vi "TAT_PLC_Data_read_BOLLEAN_St2.vi"(7 "Enum":enum16{"Read", "Write"}(ring), 8 "error in (no error)":errorcluster, 10 "Array":bool[](array[boolean])) -> (0 "error out":errorcluster, 2 "Array 2":bool[](array[boolean]))   [LabVIEW 2017]
panel:
  # "STATION 2"
  # "SCAN BYPASS---2598\nRQS TO TCO READ SCAN DATA \n\nCYCLE START (RUNNING CYCLE)\nCYCLE STOP\nCYCLE COMPLETE\nby pass station 1 Bit --45325\nStation 1 valid BIT\nPOWER FOLD CURENT M603---2651\nGLASS ACTUATOR CURANT 1 MA\nGLASS ACTUATOR CURANT 2 MA\n\n\nGLASS PUL TEST\nSKY \nGROUND\nINTERNAL(DEG)\nEXTERNAL(DEG)\n GASKET PRESENT SENSOR 1 D1811\n GASKET PRESENT SENSOR 2\n PY1B & HBC LH PART VERIFICATION SENSOR\n PY1B & HBC RH PART VERIFICATION SENSOR\n PY1B LHD RH PART SENSOR\n PY1B LHD LH PART SENSOR\n RAREJECTION BIN\n PRINT LABEL PICKUP"
  # "CONTROL PROCESS TO  LABVIEW from PLC"
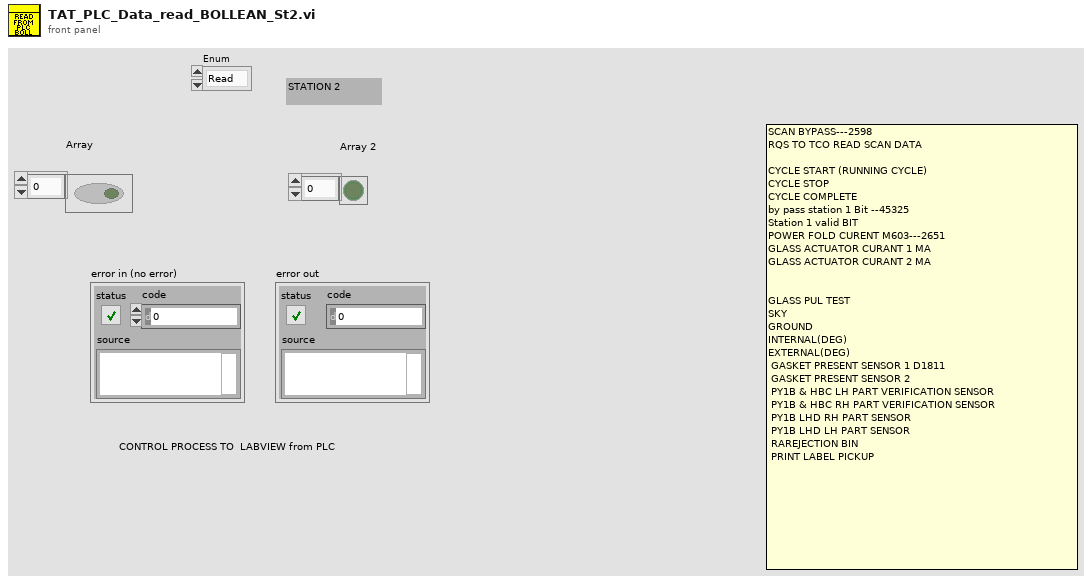
[diagram p1: front panel]
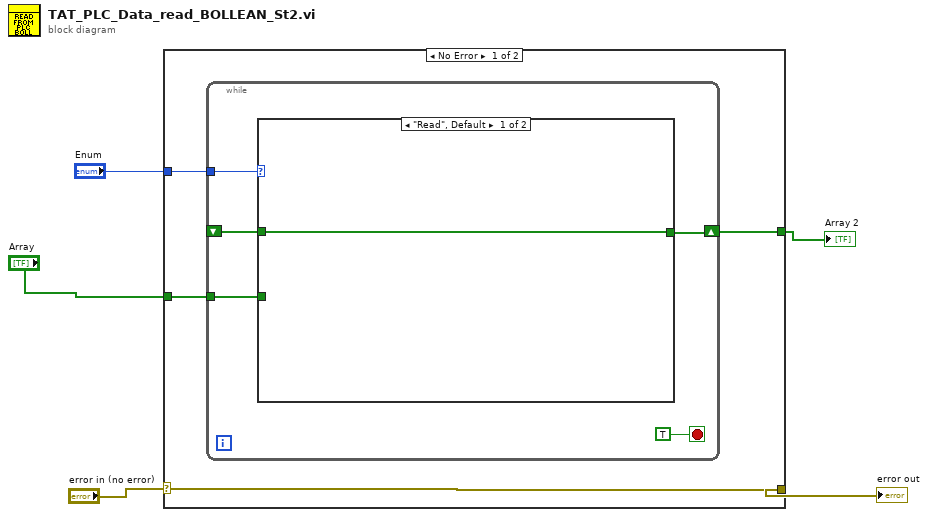
[diagram p0: block diagram]
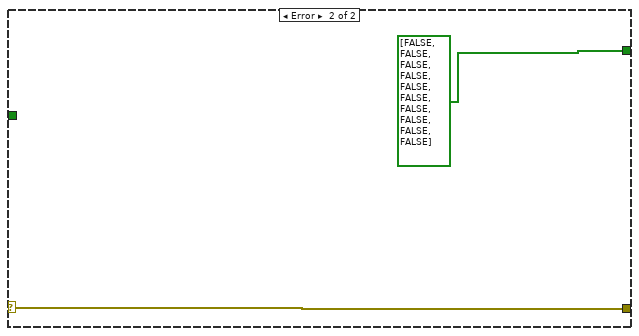
[diagram p3: hidden frame]
diagram:
  n1 = case shown="No Error" "error in (no error)" {
    selector: "error in (no error)" -> [w6 w18]
    tunnel: [w6 w18] -> w5
    tunnel: "Enum" -> [w9 _]
    tunnel: "Array" -> [w8 _]
    tunnel: [w7 bool[] [FALSE, FALSE, FALSE, FALSE, FALSE, FALSE, FALSE, FALSE, FALSE, FALSE]] -> w1
    frame No Error {
      n2 = while {
        tunnel: w9 -> [w13]
        shift-right: [w10] -> w7
        shift-left: _ -> [w11]
        tunnel: w8 -> [w12]
        stop <- TRUE stop-if-true
        n3 = case shown="\"Read\", Default" w13 {
          tunnel: w12 -> [_ w16]
          tunnel: [w15 w16] -> w10
          tunnel: w11 -> [w15 _]
          frame "Read", Default {
          }
          frame "Write" {
          }
        }
      }
    }
    frame Error {
    }
  }
  "error out" <- w5
  "Array 2" <- w1
